vi "Test_NIAI.vi"() -> ()   [LabVIEW 2019]
uses:
  Set_NIAI.ctl
  cnt_NIAI.ctl
  _ctrl/rw.ctl
panel:
  in  "cDAQ 9221 Config":T1={"input terminal"=10083, "minimum value"=-10.0, "maximum value"=10.0, "number of samples"=1000, "rate"=10000.0, "sample mode"=10123, "physical channels"="cDAQ9185-213AA55Mod3/ai0"} {"sample mode" items=["Finite Samples"=10178, "Continuous Samples"=10123, "Hardware Timed Single Point"=12522]; "rate" format="%0.2f"; "maximum value" format="%^.2e"; "minimum value" format="%^.2e"; "input terminal" items=["default"=-1, "RSE"=10083, "NRSE"=10078, "Differential"=10106, "Pseudodifferential"=12529]}
  out "Waveform Graph":waveform(dbl)[](graph)=[{"t0"=timestamp(3809335648.7877665 s since 1904-01-01), "dt"=9.999999999999999e-05, "Y"=array[1000 elements], "attributes"=variant("NI_ChannelName"=variant(string "cDAQ9185-213AA55Mod3/ai0"), "NI_UnitDescription"=variant(string "Volts"))}]
  in  "stop":bool
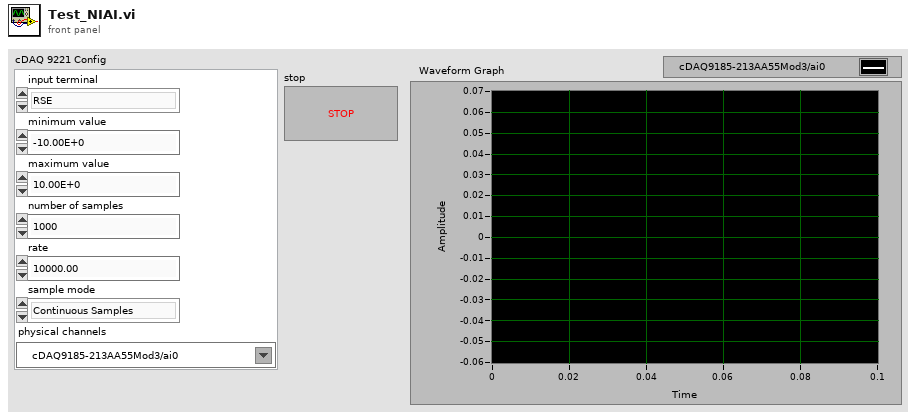
[diagram p1: front panel]
types:
  T1 = typedef "Set_NIAI.ctl" = cluster{"input terminal":i32, "minimum value":dbl, "maximum value":dbl, "number of samples":i32, "rate":dbl, "sample mode":i32, "physical channels":tag}
  T2 = typedef "cnt_NIAI.ctl" = enum16{"Open", "Read", "Close"}
  T3 = typedef "rw.ctl" = enum16{"read", "write"}
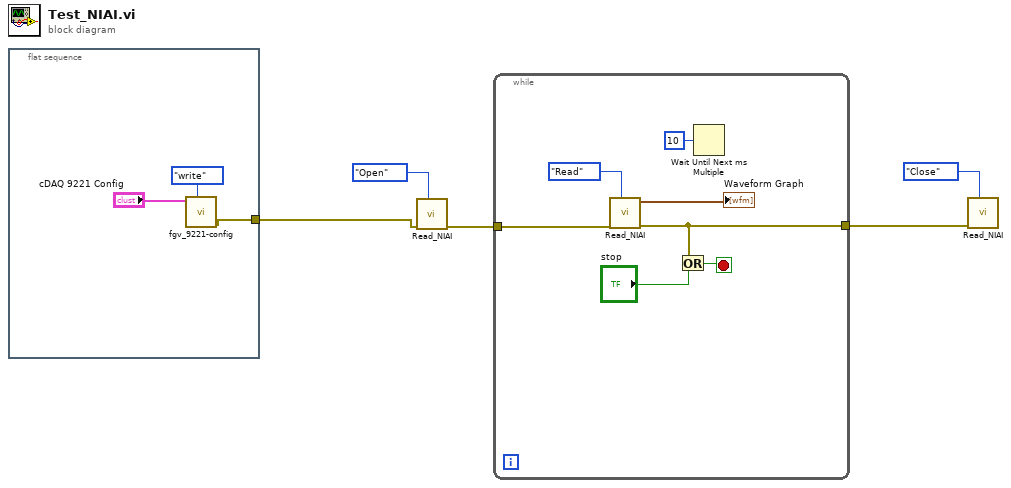
[diagram p0: block diagram]
diagram:
  n1 = flat-sequence {
    tunnel: [w7] -> w1
    frame #0 {
      n2 = call "fgv_9221-config.vi"("cmd"=rw."write", "cDAQ 9221 Config"="cDAQ 9221 Config") -> ("error out"=w7:errorcluster)  [unwired: 8 in, 1 out]
    }
  }
  n3 = call "Read_NIAI.vi"("cnt"=cnt_NIAI."Open", "error in"=w1) -> ("error out"=w3:errorcluster)  [unwired: 7 in, 2 out]
  n4 = while {
    tunnel: w3 -> [w14]
    tunnel: [w13] -> w2
    stop <- w11 stop-if-true
    n5 = call "Read_NIAI.vi"("cnt"=cnt_NIAI."Read", "error in"=w14) -> ("error out"=w13:errorcluster, "data"=→"Waveform Graph":waveform(dbl)[])  [unwired: 7 in, 1 out]
    n6 = Or(x=w13, y="stop") -> (x .or. y?=w11:bool)
    n7 = Wait Until Next ms Multiple(millisecond multiple=u32 10) -> ()  [unwired: 1 out]
  }
  n8 = call "Read_NIAI.vi"("cnt"=cnt_NIAI."Close", "error in"=w2) -> ()  [unwired: 7 in, 3 out]
